vi "IBM4_Diff_Read(IN).vi"(7 "Number":i32=10, 8 "error in":errorcluster, 9 "Neg-Chan":i32=1, 10 "Pos-Chan":i32, 11 "COM resource in":refnum<visa-resource-name>="COM9") -> (0 "error out":errorcluster, 2 "array":i32[](array[numeric]), 3 "COM resource out":refnum<visa-resource-name>)   [LabVIEW 2021, in "IBM4.lvlib"]
doc: "This VI interfaces with the IBM4 to perform a differential read operation.\n\nThe input channels must be between 0 and 4, and the number of readings should be greater than zero. At some point the number of reading will be too high and will cause a timeout error. This should only happen for numbers larger than 10000. The output will be an array of integer values.\n\nAlternate read operations exist covering binary or floating point, single reading, multiple readings, and an average of multiple readings (floating point only)."
uses:
  IBM4.lvlib
  <vilib>/Instr/_visa.llb/VISA Configure Serial Port (Instr).vi
  <vilib>/regexp/Match Regular Expression.xnode
panel:
  out "error out 2":errorcluster
  out "read buffer":string
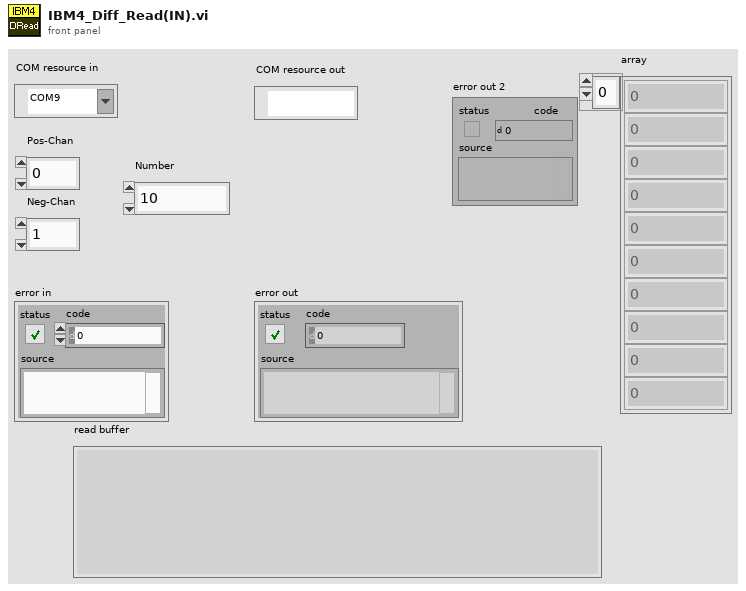
[diagram p1: front panel]
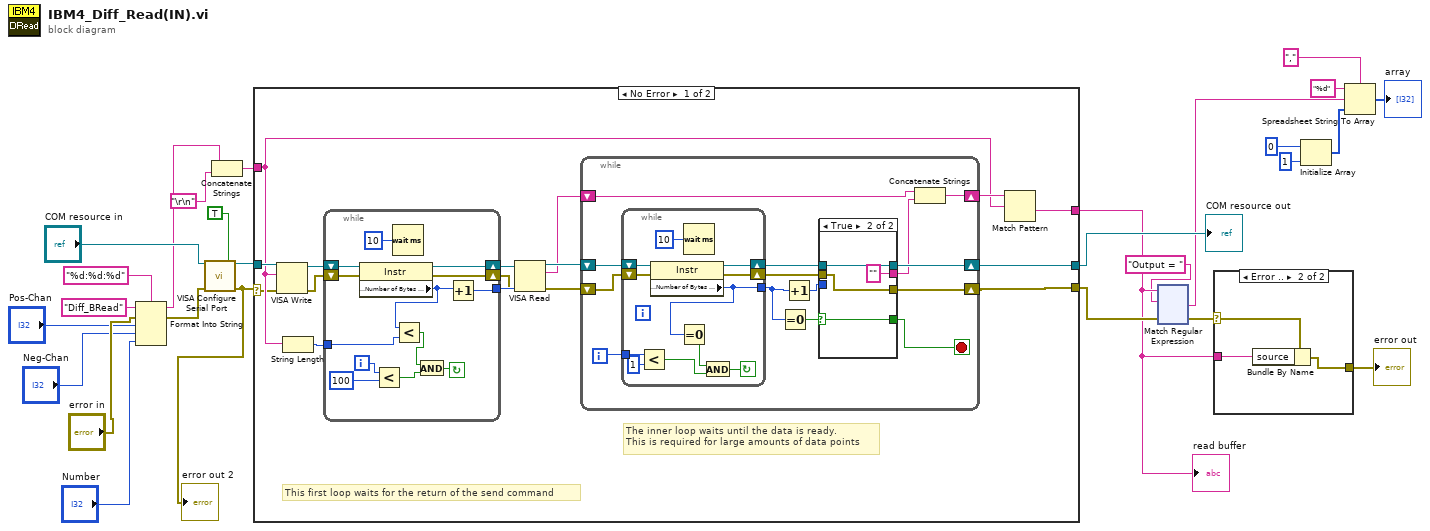
[diagram p0: block diagram]
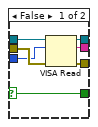
[diagram p3: hidden frame]
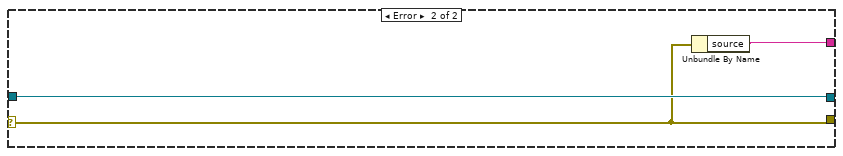
[diagram p4: hidden frame]
diagram:
  n1 = Format Into String(format string="%d:%d:%d", initial string="Diff_BRead", error in="error in", "Pos-Chan", "Neg-Chan", "Number") -> (resulting string=w16:string, error out=w23:errorcluster)
  n2 = call-poly "VISA Configure Serial Port"("VISA resource name"="COM resource in", "Enable Termination\nChar (T)"=TRUE ("Enable Termination\nChar (T)"), "error in (no error)"=w23) -> ("VISA resource name out"=w20:refnum<visa-resource-name>, "error out"=w19:errorcluster)  [unwired: 11 in]
  "error out 2" <- w19
  n3 = Concatenate Strings(w16, "\r\n") -> (w15:string)
  n4 = case shown="No Error" w19 {
    selector: w19 -> [w30 w93]
    tunnel: w20 -> [w43 w95]
    tunnel: [w29 w93] -> w5
    tunnel: [w41 w94] -> w3
    tunnel: w15 -> [w40 _]
    tunnel: [w28 w95] -> w18
    frame No Error {
      # "The inner loop waits until the data is ready.\nThis is required for large amounts of data points"
      # "This first loop waits for the return of the send command"
      n5 = VISA Write(VISA resource name=w43, write buffer=w40, error in (no error)=w30) -> (VISA resource name out=w39:refnum<visa-resource-name>, error out=w38:errorcluster)  [unwired: 1 out]
      n6 = String Length(string=w40) -> (length=w31:i32)
      n7 = while {
        tunnel: [w45] -> w36
        shift-right: [w55] -> w37
        shift-left: w39 -> [w56]
        shift-right: [w53] -> w35
        shift-left: w38 -> [w54]
        tunnel: w31 -> [w51]
        i -> [w46]
        stop <- w49 continue-if-true
        n8 = property class="Instr"(reference=w56, error in=w54) -> (reference out=w55:refnum<visa-resource-name>, error out=w53:errorcluster, "Serial Settings:Number of Bytes at Serial Port"=w44:u32)
        n9 = Less?(x=w46, y=100) -> (x < y?=w48:bool)
        n10 = Wait (ms)(milliseconds to wait=u32 10) -> ()  [unwired: 1 out]
        n11 = Less?(x=w44, y=w51) -> (x < y?=w47:bool)
        n12 = And(x=w47, y=w48) -> (x .and. y?=w49:bool)
        n13 = Increment(x=w44) -> (x+1=w45:u32)
      }
      n14 = VISA Read(VISA resource name=w37, byte count=w36, error in (no error)=w35) -> (VISA resource name out=w34:refnum<visa-resource-name>, read buffer=w32:string, error out=w33:errorcluster)  [unwired: 1 out]
      n15 = while {
        shift-right: [w70] -> w28
        shift-left: w34 -> [w68]
        shift-right: [w69] -> w29
        shift-left: w33 -> [w66]
        shift-right: [w64] -> w42
        shift-left: w32 -> [w62]
        i -> [w61]
        stop <- w57 stop-if-true
        n16 = while {
          tunnel: [w87] -> w60
          shift-right: [w91] -> w67
          shift-left: w68 -> [w92]
          shift-right: [w89] -> w65
          shift-left: w66 -> [w90]
          tunnel: w61 -> [w86]
          stop <- w84 continue-if-true
          n17 = Less?(x=w86, y=1) -> (x < y?=w83:bool)
          n18 = property class="Instr"(reference=w92, error in=w90) -> (reference out=w91:refnum<visa-resource-name>, error out=w89:errorcluster, "Serial Settings:Number of Bytes at Serial Port"=w87:u32)
          n19 = Equal To 0?(x=w87) -> (x = 0?=w82:bool)
          n20 = Wait (ms)(milliseconds to wait=u32 10) -> ()  [unwired: 1 out]
          n21 = And(x=w82, y=w83) -> (x .and. y?=w84:bool)
        }
        n22 = Equal To 0?(x=w60) -> (x = 0?=w58:bool)
        n23 = Increment(x=w60) -> (x+1=w59:u32)
        n24 = case shown="True" w58 {
          selector: w58 -> [w71 w80]
          tunnel: [w77 w81] -> w70
          tunnel: [w76 w79] -> w69
          tunnel: w67 -> [w75 w81]
          tunnel: w65 -> [w74 w79]
          tunnel: [w73 "" ("read buffer")] -> w63
          tunnel: w59 -> [w72 _]
          tunnel: [w71 w80] -> w57
          frame False {
            n25 = VISA Read(VISA resource name=w75, byte count=w72, error in (no error)=w74) -> (VISA resource name out=w77:refnum<visa-resource-name>, read buffer=w73:string, error out=w76:errorcluster)  [unwired: 1 out]
          }
          frame True {
          }
        }
        n26 = Concatenate Strings(w62, w63) -> (w64:string)
      }
      n27 = Match Pattern(string=w42, regular expression=w40) -> (after substring=w41:string)  [unwired: 1 in, 3 out]
    }
    frame Error {
      n28 = Unbundle By Name(w93) -> ("source"=w94:string)
    }
  }
  "COM resource out" <- w18
  "read buffer" <- w3
  n29 = xnode "Match Regular Expression"("input string"=w3, "regular expression"="Output = " ("format string"), "error in"=w5) -> ("after match"=w1:string, "error out"=w4:errorcluster)  [unwired: 3 in, 3 out]
  n30 = case shown="Error .." w4 {
    selector: w4 -> [w96 w99]
    tunnel: [w96 w97] -> w14
    tunnel: w3 -> [_ w98]
    frame No Error {
    }
    frame Error {
      n31 = Bundle By Name(cluster=w99, "source"=w98) -> (w97:errorcluster)
    }
  }
  "error out" <- w14
  n32 = Initialize Array(0, 1 ("dimension size")) -> (w10:i32[])
  n33 = Spreadsheet String To Array(delimiter (Tab)=",", format string="%d", spreadsheet string=w1, array type (2D Dbl)=w10) -> (array=→"array":i32[])
